vi "Master Setup Read Write RT Update Errors.vi"(7 "RT Update Timestamp":timestamp, 8 "Reset":bool, 9 "Read (F) Write (T)":bool, 10 "Pattern Label":T1 items=["Channel Setup (0)", "PID Setup (1)", "Filter Setup (2)", "~Reserved Old CAN Msgs (3)", "~Reserved Old CAN1 (4)", "~Reserved Old CAN2 (5)", "Digital Inputs Setup (6)", "Digital Outputs Setup (7)", "Logging 1 Setup (8)", "Logging 2 Setup (9)", "Logging 3 Setup (10)", "Setpoint Setup (11)", "Test Series Setup (12)", "Graph Setup (13)", "System Configure (14)", "Header (15)", "Profile Manager (16)", "Post-Mortem Logging (17)", "High-Speed Data (18)", "Statistic Channel Setup (19)", "Ramp Channel Setup (20)", "ETAS INCA Channel Setup (21)", "ETC ECCS Transducer Setup (22)", "ETC ECCS Test Setup (23)", "AVL AK Smoke Meter Setup (24)", "Triggers Setup (25)", "Alarm Limits Setup (26)", "YKWT1 Measurement (27)", "YKWT1 Instrument (28)", "Auto File Settings (29)", "Playback File Setting (30)", "UUT Constants (31)", "UPS Setup (32)", "Differential Channel Setup (33)", "Integral Channel Setup (34)", "Signal Channel Setup (35)", "Calibration Setup (36)", "BNC Setup (37)", "ASAP3 Setup (38)", "Chassis Force Calculations (39)", "Chassis Teststand Losses (40)", "Chassis Vehicle Losses (41)", "Formula Channels (42)", "ASAP3 Map Coords Setup (43)", "Digital Controls Setup (44)", "Push Buttons Setup (45)", "Sliders Setup (46)", "~Reserved~ (47)", "Email Setup (48)", "Timer Setup (49)", "Unit Conversion Setup (50)", "Visible Channels (51)", "Main Display Setup (52)", "Message Display Setup (53)", "Input Display Setup (54)", "Unico Parameter Downloads (55)", "Flow Meter Setup (56)", "Channel Zero Offset (57)", "YKWT2 Measurement (58)", "YKWT2 Instrument (59)", "~Reserved Old CAN3 (60)", "CAS Setup (61)", "Accumulation Channel Setup (62)", "Valvetrain Dynamics Setup (63)", "CCP Setup (64)", "System Log Setup (65)", "Throttle Controller (66)", "RE Shifter (67)", "Main Display (68)", "~Reserved~ (69)", "FlexRay (70)", "YKWT3 Measurement (71)", "YKWT3 Instrument (72)", "CAN XNET API (73)"], 11 "Error Status":bool) -> (1 "Update Timestamp":timestamp[](array[timestamp]), 2 "All Real-Time Update Successful?":bool, 3 "Real-Time Update Status (out)":bool[](array[boolean]))   [LabVIEW 2017]
uses:
  Master Setup Pattern Enum.ctl
  Event Log PC/Event Control.ctl
panel:
  out "error out":errorcluster
  in  "error in (no error)":errorcluster
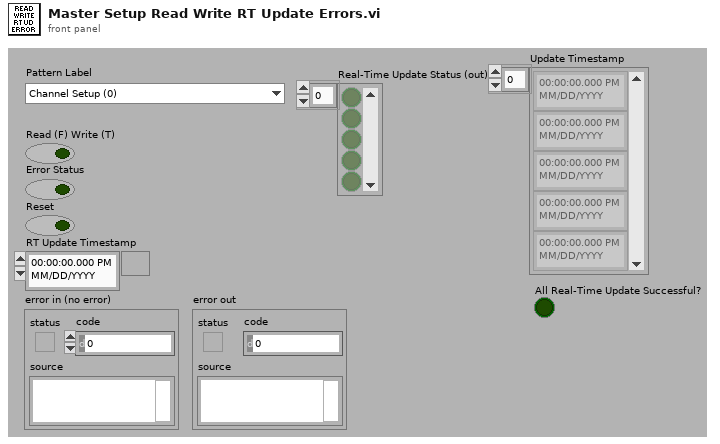
[diagram p1: front panel]
types:
  T1 = typedef "Master Setup Pattern Enum.ctl" = i32
  T2 = typedef "Event Control.ctl" = cluster{"Task":string, "Pass/Fail":string, "Module No.":i32, "Module":string, "Description":string}
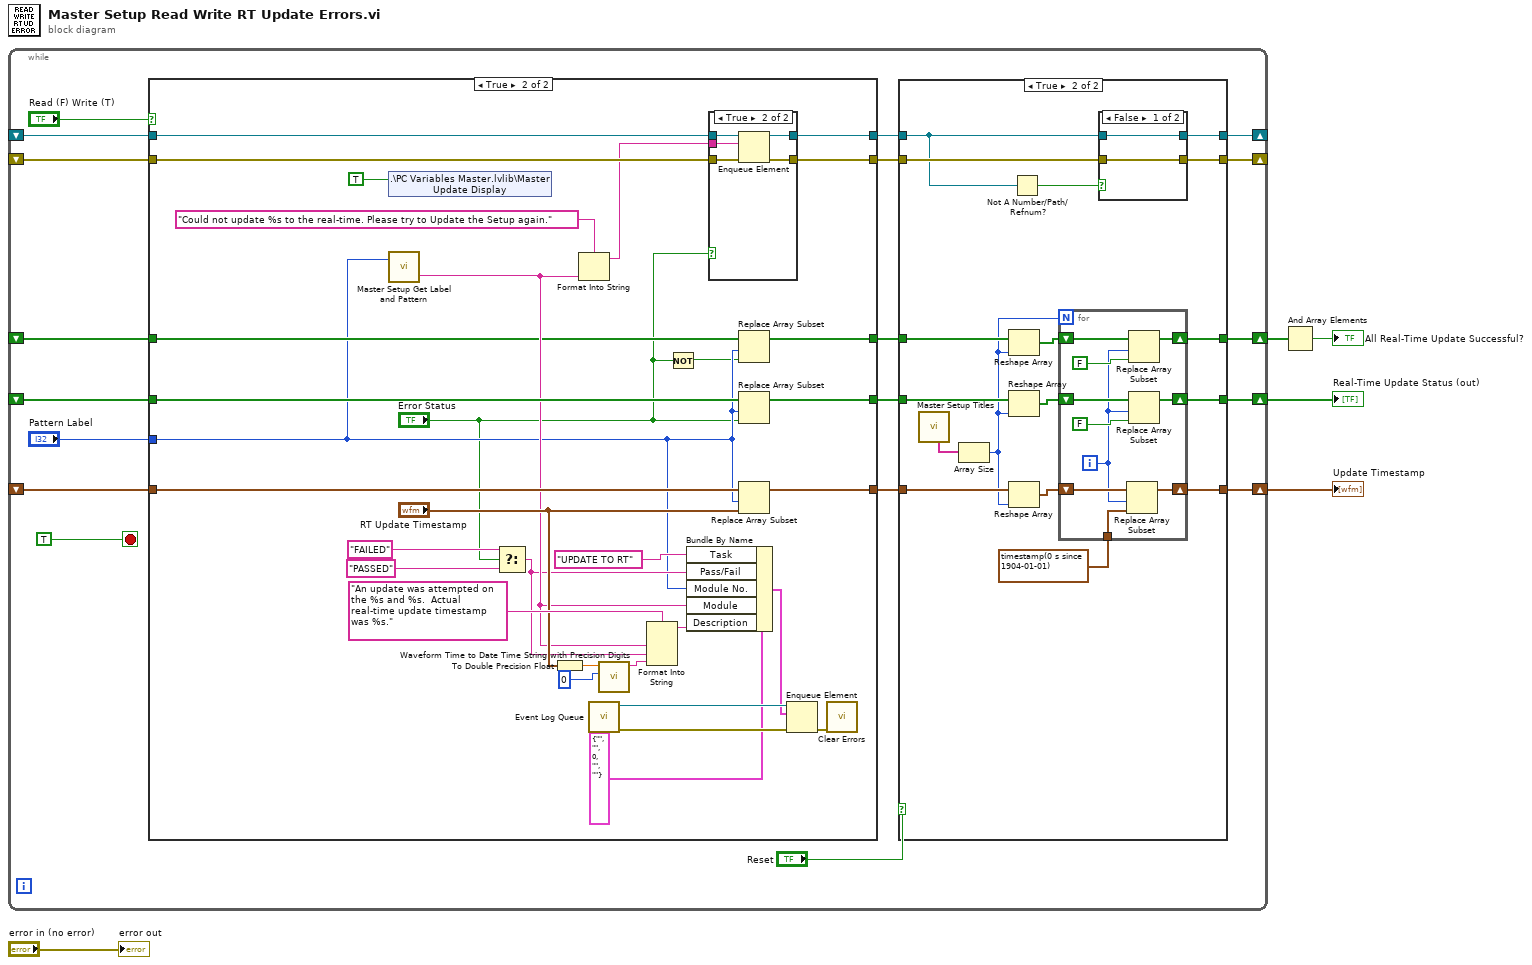
[diagram p0: block diagram]
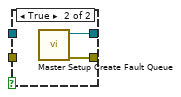
[diagram p5: hidden frame]
diagram:
  n1 = while {
    shift-right: [w23] -> w3
    shift-left: _ -> [w22]
    shift-right: [w20] -> _
    shift-left: _ -> [w18]
    shift-right: [w19] -> _
    shift-left: _ -> [w16]
    shift-right: [w10] -> w4
    shift-left: _ -> [w9]
    shift-right: [w8] -> w2
    shift-left: _ -> [w6]
    stop <- TRUE stop-if-true
    n2 = case shown="True" "Read (F) Write (T)" {
      tunnel: [w29 w61] -> w21
      tunnel: w22 -> [w29 w60]
      tunnel: "Pattern Label" -> [_ w32]
      tunnel: w18 -> [w28 w58]
      tunnel: [w28 w57] -> w17
      tunnel: w16 -> [w27 w56]
      tunnel: [w27 w55] -> w15
      tunnel: [w26 w52] -> w11
      tunnel: w9 -> [w26 w51]
      tunnel: [w25 w34] -> w7
      tunnel: w6 -> [w25 w33]
      frame False {
      }
      frame True {
        n3 = shared-variable ".\\PC Variables Master.lvlib\\Master Update Display"(TRUE ("Master Update Display")) -> ()  [unwired: 1 in, 1 out]
        n4 = call "Master Setup Get Label and Pattern.vi"("Master Setup Patten Enum"=w32) -> ("Pattern Label"=w42:string)  [unwired: 1 in, 1 out]
        n5 = Select(t="FAILED" ("[Date/Time] [Fault Status] [Fault Type] ... [Channel Name] ... [Value] ... [Limit]"), s="Error Status", f="PASSED" ("[Date/Time] [Fault Status] [Fault Type] ... [Channel Name] ... [Value] ... [Limit]")) -> (s? t:f=w35:string)
        n6 = To Double Precision Float(number="RT Update Timestamp") -> (double precision float=w38:dbl)
        n7 = Format Into String(format string="Could not update %s to the real-time. Please try to Update the Setup again." ("[Date/Time] [Fault Status] [Fault Type] ... [Channel Name] ... [Value] ... [Limit]"), w42) -> (resulting string=w53:string)  [unwired: 2 in, 1 out]
        n8 = call "Event Log Queue.vi"() -> ("error out"=w45:errorcluster, "Event Queue"=w46:refnum<queue>)  [unwired: 6 in]
        n9 = call "Waveform Time to Date Time String with Precision Digits.vi"("Number of digits of precision (4)"=u32 0, "t0"=w38) -> ("String"=w37:string)  [unwired: 9 in]
        n10 = Format Into String(format string="An update was attempted on the %s and %s.  Actual real-time update timestamp was %s." ("[Date/Time] [Fault Status] [Fault Type] ... [Channel Name] ... [Value] ... [Limit]"), w42, w35, w37) -> (resulting string=w43:string)  [unwired: 2 in, 1 out]
        n11 = Not(x="Error Status") -> (.not. x?=w31:bool)
        n12 = Bundle By Name(cluster=T2 {"Task"="", "Pass/Fail"="", "Module No."=0, "Module"="", "Description"=""} ("element"), "Task"="UPDATE TO RT", "Pass/Fail"=w35, "Module No."=w32, "Module"=w42, "Description"=w43) -> (w39:T2)
        n13 = case shown="True" "Error Status" {
          tunnel: w58 -> [w63 w68]
          tunnel: [w63 w67] -> w57
          tunnel: w56 -> [w62 w66]
          tunnel: [w62 w65] -> w55
          tunnel: w53 -> [_ w64]
          frame False {
          }
          frame True {
            n14 = Enqueue Element(queue=w68, element=w64, error in (no error)=w66) -> (queue out=w67:refnum<queue>, error out=w65:errorcluster)  [unwired: 1 in, 1 out]
          }
        }
        n15 = Replace Array Subset(array=w33, new element=w31, index=w32) -> (w34:bool[])
        n16 = Replace Array Subset(array=w60, new element="Error Status", index=w32) -> (w61:bool[])
        n17 = Replace Array Subset(array=w51, new element="RT Update Timestamp", index=w32) -> (w52:timestamp[])
        n18 = Enqueue Element(queue=w46, element=w39, error in (no error)=w45) -> (error out=w44:errorcluster)  [unwired: 1 in, 2 out]
        n19 = call <vilib>:"Clear Errors.vi"("error in (no error)"=w44) -> ()  [unwired: 5 in, 2 out]
      }
    }
    n20 = case shown="True" "Reset" {
      tunnel: [w73 w82] -> w23
      tunnel: w21 -> [w73 w89]
      tunnel: [w72 w87] -> w20
      tunnel: w17 -> [w72 w84]
      tunnel: [w71 w86] -> w19
      tunnel: w15 -> [w71 w85]
      tunnel: w11 -> [w70 w81]
      tunnel: [w70 w79] -> w10
      tunnel: [w69 w77] -> w8
      tunnel: w7 -> [w69 w76]
      frame False {
      }
      frame True {
        n21 = call "Master Setup Titles.vi"() -> ("Sorted Setup Description"=w90:string[])  [unwired: 6 in, 5 out]
        n22 = Array Size(array=w90) -> (size(s)=w74:i32)
        n23 = Reshape Array(w76, w74) -> (w75:bool[])
        n24 = Reshape Array(w89, w74) -> (w83:bool[])
        n25 = Reshape Array(w81, w74) -> (w80:timestamp[])
        n26 = Not A Number/Path/Refnum?(number/path/refnum=w84) -> (NaN/Path/Refnum?=w88:bool)
        n27 = for {
          N: w74 -> [_]
          shift-right: [w99] -> w82
          shift-left: w83 -> [w100]
          shift-right: [w96] -> w79
          shift-left: w80 -> [w97]
          tunnel: timestamp(0 s since 1904-01-01) ("RT Update Timestamp") -> [w95]
          shift-right: [w93] -> w77
          shift-left: w75 -> [w92]
          i -> [w91]
          n28 = Replace Array Subset(array=w97, new element=w95, index=w91) -> (w96:timestamp[])
          n29 = Replace Array Subset(array=w92, new element=FALSE ("new element/subarray"), index=w91) -> (w93:bool[])
          n30 = Replace Array Subset(array=w100, new element=FALSE ("new element/subarray"), index=w91) -> (w99:bool[])
        }
        n31 = case shown="False" w88 {
          tunnel: [w102 w104] -> w87
          tunnel: w84 -> [w102 _]
          tunnel: [w101 w103] -> w86
          tunnel: w85 -> [w101 _]
          frame False {
          }
          frame True {
            n32 = call "Master Setup Create Fault Queue.vi"() -> ("error out"=w103:errorcluster, "Master Fault Queue"=w104:refnum<queue>)  [unwired: 6 in]
          }
        }
      }
    }
  }
  "Real-Time Update Status (out)" <- w3
  "Update Timestamp" <- w4
  n33 = And Array Elements(Boolean array=w2) -> (logical AND=→"All Real-Time Update Successful?":bool)
  "error out" <- "error in (no error)"
